vi "AlliGator Create Gate Image v2.vi"(0 "Dataset Images in":T6, 1 "Init?":bool, 2 "Prefix":string, 7 "Current Gate":i32, 9 "Gate Name":string, 11 "error in (no error)":errorcluster, 12 "Image Characteristics":T2 {"Calibration"."Y Step" format="%.2f"; "Calibration"."X Step" format="%.2f"; "Image Type" items=["Grayscale (U8)", "Grayscale (I16)", "Grayscale (SGL)", "Complex (CSG)", "RGB (U32)", "HSL (U32)", "RGB (U64)", "Grayscale (U16)"]}, 13 "Background Dataset":bool) -> (3 "Init?":bool, 4 "Dataset Images out":T6, 8 "New Gate Image Refnum":T1, 10 "Buffer Image available?":bool, 14 "Number of Created Images":i32, 15 "error out":errorcluster)   [LabVIEW 2021, in "AlliGator Files.lvlib"]
doc: "Creates image structure(s) for the new loaded gate, if needed."
uses:
  AlliGator Files.lvlib
  AlliGator Gate Image Set.ctl
  <vilib>/vision/Image Controls.llb/IMAQ Image.ctl
  Image/Image Characteristics.ctl
  Image/Image.lvlib
panel:
  # "see the AlliGator License on the block diagram (Ctrl+E or Window:Show Block Diagram)"
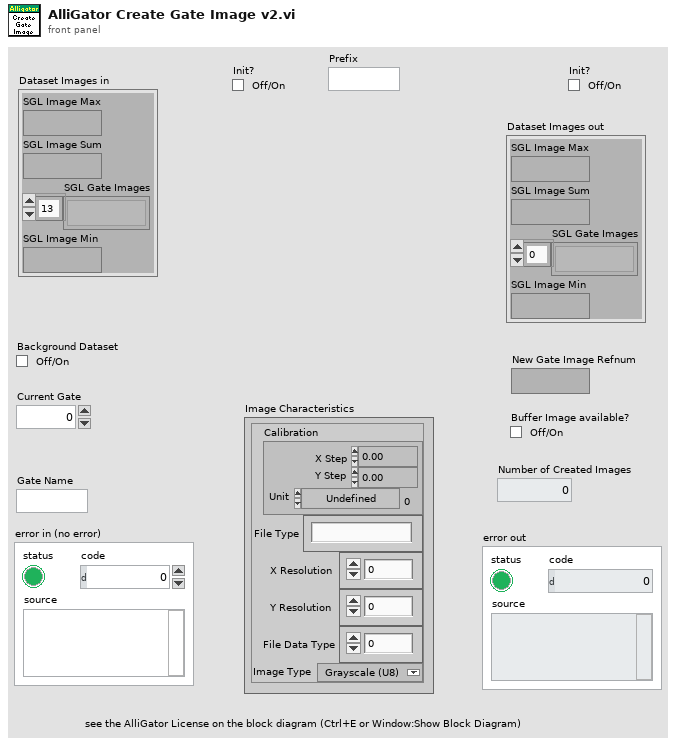
[diagram p1: front panel]
types:
  T1 = typedef "IMAQ Image.ctl" = refnum<image>
  T2 = typedef "Image.lvlib/Image Characteristics.ctl" = cluster{"Calibration":T3, "File Type":string, "X Resolution":i32, "Y Resolution":i32, "File Data Type":i32, "Image Type":T5}
  T3 = typedef "Simple Grid Descriptor" = cluster{"X Step":sgl, "Y Step":sgl, "Unit":T4}
  T4 = typedef "Image Unit" = enum32{"Undefined", "Angström", "Micrometer", "Millimeter", "Centimeter", "Meter", "Kilometer", "Microinch", "Inch", "Feet", "Nautical miles", "Standard miles", "Steps"}
  T5 = typedef "Image Type" = u32
  T6 = typedef "AlliGator Files.lvlib/AlliGator Gate Image Set.ctl" = cluster{"SGL Image Max":T1, "SGL Image Sum":T1, "SGL Gate Images":T1[], "SGL Image Min":T1}
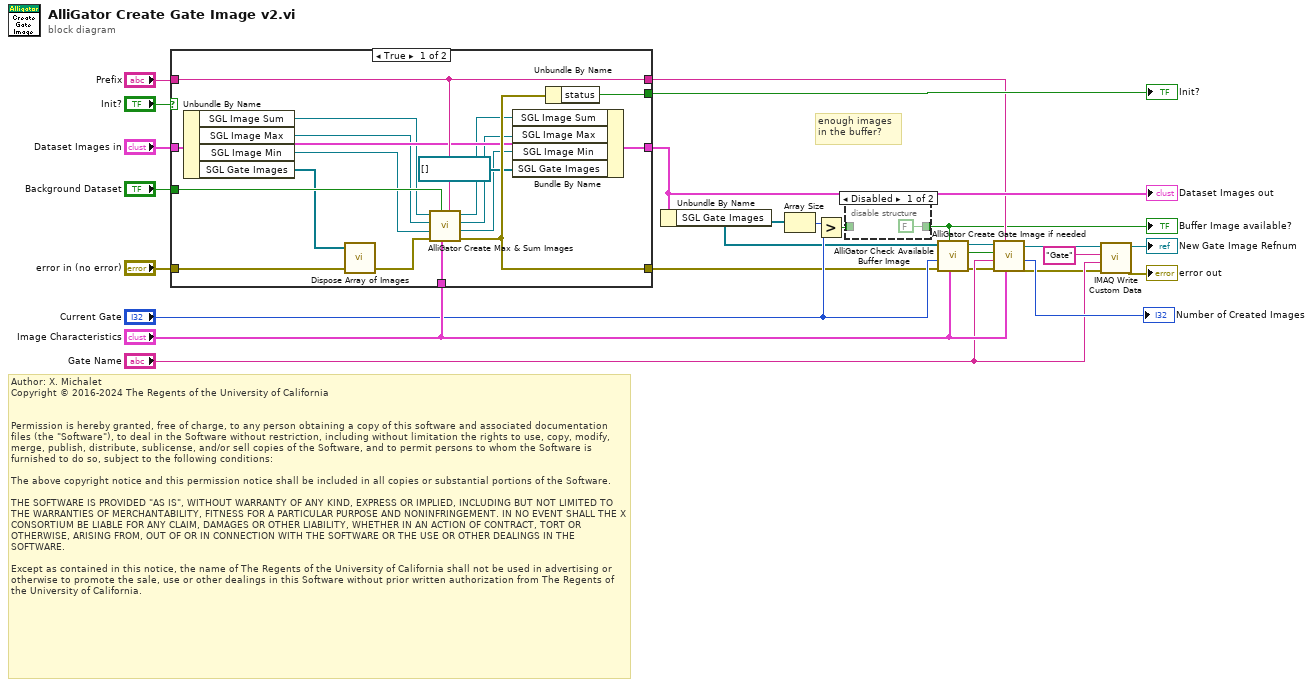
[diagram p0: block diagram]
diagram:
  # "Author: X. Michalet\nCopyright © 2016-2024 The Regents of the University of California\n \n\nPermission is hereby granted, free of charge, to any person obtaining a copy of this software and associated documentation files (the \"Software\"), to deal in the Software without restriction, including without limitation the rights to use, copy, modify, merge, publish, distribute, sublicense, and/or sell copies of the Software, and to permit persons to whom the Software is furnished to do so, subject to the following conditions:\n\nThe above copyright notice and this permission notice shall be included in all copies or substantial portions of the Software.\n\nTHE SOFTWARE IS PROVIDED \"AS IS\", WITHOUT WARRANTY OF ANY KIND, EXPRESS OR IMPLIED, INCLUDING BUT NOT LIMITED TO THE WARRANTIES OF MERCHANTABILITY, FITNESS FOR A PARTICULAR PURPOSE AND NONINFRINGEMENT. IN NO EVENT SHALL THE X CONSORTIUM BE LIABLE FOR ANY CLAIM, DAMAGES OR OTHER LIABILITY, WHETHER IN AN ACTION OF CONTRACT, TORT OR OTHERWISE, ARISING FROM, OUT OF OR IN CONNECTION WITH THE SOFTWARE OR THE USE OR OTHER DEALINGS IN THE SOFTWARE.\n\nExcept as contained in this notice, the name of The Regents of the University of California shall not be used in advertising or otherwise to promote the sale, use or other dealings in this Software without prior written authorization from The Regents of the University of California."
  # "enough images in the buffer?"
  n1 = case shown="True" "Init?" {
    selector: "Init?" -> [_ w46]
    tunnel: "error in (no error)" -> [w37 w45]
    tunnel: [w39 w46] -> w8
    tunnel: [w40 w45] -> w9
    tunnel: "Background Dataset" -> [w42 _]
    tunnel: "Image Characteristics" -> [w41 _]
    tunnel: "Prefix" -> [w34 w43]
    tunnel: "Dataset Images in" -> [w33 w44]
    tunnel: [w35 w44] -> w5
    tunnel: [w34 w43] -> w3
    frame True {
      n2 = Unbundle By Name(w33) -> ("SGL Image Sum"=w31:T1, "SGL Image Max"=w30:T1, "SGL Image Min"=w29:T1, "SGL Gate Images"=w36:T1[])
      n3 = call "Dispose Array of Images.vi"("Array of Images"=w36, "error in (no error)"=w37) -> ("error out"=w38:errorcluster)  [unwired: 7 in]
      n4 = call "AlliGator Create Max & Sum Images.vi"("Prefix"=w34, "Image Characteristics"=w41, "Image Type"=w42, "Error In"=w38, "Image Min"=w29, "Image Max"=w30, "Image Sum"=w31) -> ("Error Out"=w40:errorcluster, "Image Min"=w26:T1, "Image Max"=w27:T1, "Image Sum"=w28:T1)  [unwired: 1 in]
      n5 = Bundle By Name(cluster=w33, "SGL Image Sum"=w28, "SGL Image Max"=w27, "SGL Image Min"=w26, "SGL Gate Images"=T1[] []) -> (w35:T6)
      n6 = Unbundle By Name(w40) -> ("status"=w39:bool)
    }
    frame False {
    }
  }
  "Dataset Images out" <- w5
  "Init?" <- w8
  n7 = Unbundle By Name(w5) -> ("SGL Gate Images"=w4:T1[])
  n8 = Array Size(array=w4) -> (size(s)=w10:i32)
  n9 = Greater?(x=w10, y="Current Gate") -> (0:w2:bool)
  n10 = disable-structure shown="Disabled" {
    disable-tunnel: w2 -> [_ w48]
    disable-tunnel: [FALSE w48] -> w1
    frame Disabled {
    }
    frame Enabled {
    }
  }
  "Buffer Image available?" <- w1
  n11 = call "AlliGator Check Available Buffer Image.vi"("Image Characteristics"="Image Characteristics", "Buffer Image available?"=w1, "error in (no error)"=w9, "Current Gate"="Current Gate", "Image Buffer"=w4) -> ("error out"=w12:errorcluster, "Image Reused?"=w14:bool, "Gate Image"=w13:T1)  [unwired: 3 in, 1 out]
  n12 = call "AlliGator Create Gate Image if needed.vi"("Image Characteristics"="Image Characteristics", "Prefix String"=w3, "error in (no error)"=w12, "Gate ID"="Gate Name", "Image Reused?"=w14, "Gate Image"=w13) -> ("error out"=w18:errorcluster, "Number of Created Images"=→"Number of Created Images":i32, "Gate Image"=w15:T1)  [unwired: 2 in, 1 out]
  n13 = call "IMAQ Write Custom Data"("error in (no error)"=w18, "Custom Data In"="Gate Name", "Key"="Gate", "Image"=w15) -> ("error out"=→"error out":errorcluster, "Image Out"=→"New Gate Image Refnum":T1)  [unwired: 6 in]
